vi "Format Data to Save.vi"(5 "Sections":i32=100, 6 "FilePath":path, 7 "LoopBeginWait(ms)":u32=100, 9 "Time":dbl[](array[numeric]), 11 "Data":dbl[][](array[numeric])) -> ()   [LabVIEW 2018]
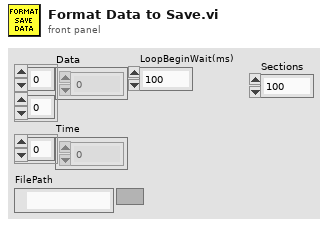
[diagram p1: front panel]
types:
  T1 = enum16{"open", "replace", "create", "open or create", "replace or create", "replace or create with confirmation"}
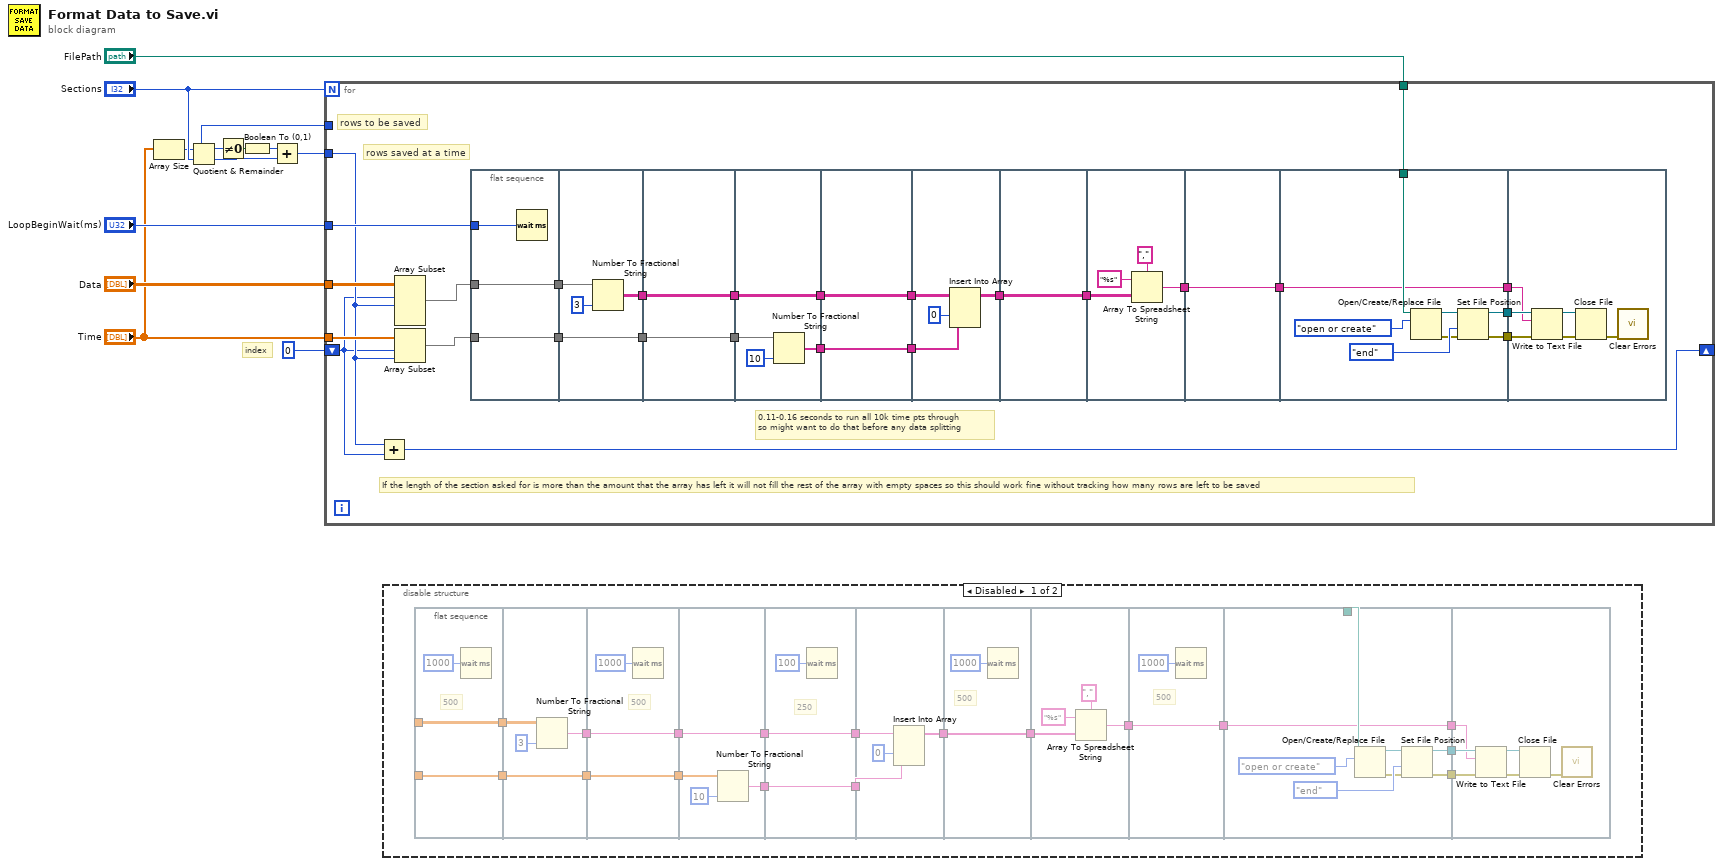
[diagram p0: block diagram]
diagram:
  # "index"
  n1 = Array Size(array="Time") -> (size(s)=w2:i32)
  n2 = Quotient & Remainder(x=w2, y="Sections") -> (x-y*floor(x/y)=w4:i32, floor(x/y)=w5:i32)
  n3 = Not Equal To 0?(x=w4) -> (x != 0?=w7:bool)
  n4 = Boolean To (0,1)(Boolean=w7) -> (0, 1=w6:i16)
  n5 = Add(x=w6, y=w5) -> (x+y=w3:i32)
  n6 = for {
    N: "Sections" -> [_]
    tunnel: "Time" -> [w18]
    tunnel: "Data" -> [w19]
    tunnel: "FilePath" -> [w21]
    tunnel: "LoopBeginWait(ms)" -> [w20]
    tunnel: w3 -> [w14]
    tunnel: w2 -> [_]
    shift-right: [w15] -> _
    shift-left: 0 -> [w13]
    # "rows saved at a time"
    # "rows to be saved"
    # "If the length of the section asked for is more than the amount that the array has left it will not fill the rest of the array with empty spaces so this should work fine without tracking how many rows are left to be saved"
    # "0.11-0.16 seconds to run all 10k time pts through\nso might want to do that before any data splitting"
    n7 = Add(x=w14, y=w13) -> (x+y=w15:i32)
    n8 = Array Subset(array=w19, index (row)=w13, length (row)=w14) -> (w16:dbl[][])  [unwired: 2 in]
    n9 = Array Subset(array=w18, index=w13, length=w14) -> (w17:dbl[])
    n10 = flat-sequence {
      tunnel: w16 -> [w40]
      tunnel: w17 -> [w41]
      tunnel: [w41] -> w38
      tunnel: [w40] -> w37
      tunnel: w20 -> [w39]
      tunnel: w38 -> [w43]
      tunnel: w37 -> [w44]
      tunnel: [w43] -> w36
      tunnel: [w42] -> w35
      tunnel: [w47] -> w34
      tunnel: w36 -> [w47]
      tunnel: w35 -> [w46]
      tunnel: [w46] -> w33
      tunnel: w34 -> [w50]
      tunnel: [w49] -> w32
      tunnel: [w48] -> w31
      tunnel: w33 -> [w48]
      tunnel: w32 -> [w53]
      tunnel: w31 -> [w52]
      tunnel: [w52] -> w30
      tunnel: [w53] -> w29
      tunnel: w30 -> [w56]
      tunnel: w29 -> [w55]
      tunnel: [w54] -> w28
      tunnel: w28 -> [w58]
      tunnel: [w58] -> w27
      tunnel: w27 -> [w60]
      tunnel: [w59] -> w26
      tunnel: w26 -> [w63]
      tunnel: [w63] -> w25
      tunnel: w25 -> [w64]
      tunnel: w21 -> [w67]
      tunnel: [w66] -> w24
      tunnel: [w65] -> w23
      tunnel: [w64] -> w22
      tunnel: w24 -> [w74]
      tunnel: w23 -> [w73]
      tunnel: w22 -> [w72]
      frame #0 {
        n11 = Wait (ms)(milliseconds to wait=w39) -> ()  [unwired: 1 out]
      }
      frame #1 {
        n12 = Number To Fractional String(number=w44, precision (6)=i16 3) -> (F-format string=w42:string[][])  [unwired: 2 in]
      }
      frame #2 {
      }
      frame #3 {
        n13 = Number To Fractional String(number=w50, precision (6)=i16 10) -> (F-format string=w49:string[])  [unwired: 2 in]
      }
      frame #4 {
      }
      frame #5 {
        n14 = Insert Into Array(array=w56, index (col)=0 ("disabled index (col)"), new element=w55) -> (w54:string[][])  [unwired: 1 in]
      }
      frame #6 {
      }
      frame #7 {
        n15 = Array To Spreadsheet String(delimiter (Tab)=",", array=w60, 3:"%s" ("format string")) -> (spreadsheet string=w59:string)
      }
      frame #8 {
      }
      frame #9 {
        n16 = Open/Create/Replace File(file path (use dialog)=w67, operation (0:open)=T1."open or create") -> (refnum out=w69:refnum<file>, error out=w70:errorcluster)  [unwired: 4 in, 1 out]
        n17 = Set File Position(refnum=w69, from (0:start)=enum16{"start", "end", "current"}."end", error in=w70) -> (refnum out=w66:refnum<file>, error out=w65:errorcluster)  [unwired: 1 in]
      }
      frame #10 {
        n18 = Write to Text File(file (use dialog)=w74, text=w72, error in=w73) -> (refnum out=w76:refnum<file>, error out=w75:errorcluster)  [unwired: 1 in, 1 out]
        n19 = Close File(refnum=w76, error in=w75) -> (error out=w77:errorcluster)  [unwired: 1 out]
        n20 = call <vilib>:"Clear Errors.vi"("error in (no error)"=w77) -> ()  [unwired: 5 in, 2 out]
      }
    }
  }
  n21 = disable-structure shown="Disabled" {
    frame Disabled {
      n22 = flat-sequence {
        tunnel: _ -> [w96]
        tunnel: _ -> [w97]
        tunnel: [w97] -> w94
        tunnel: [w96] -> w93
        tunnel: w94 -> [w99]
        tunnel: w93 -> [w100]
        tunnel: [w99] -> w92
        tunnel: [w98] -> w91
        tunnel: [w104] -> w90
        tunnel: w92 -> [w104]
        tunnel: w91 -> [w102]
        tunnel: [w102] -> w89
        tunnel: w90 -> [w107]
        tunnel: [w106] -> w88
        tunnel: [w105] -> w87
        tunnel: w89 -> [w105]
        tunnel: w88 -> [w111]
        tunnel: w87 -> [w110]
        tunnel: [w110] -> w86
        tunnel: [w111] -> w85
        tunnel: w86 -> [w114]
        tunnel: w85 -> [w113]
        tunnel: [w112] -> w84
        tunnel: w84 -> [w117]
        tunnel: [w117] -> w83
        tunnel: w83 -> [w119]
        tunnel: [w118] -> w82
        tunnel: w82 -> [w123]
        tunnel: [w123] -> w81
        tunnel: w81 -> [w124]
        tunnel: _ -> [w127]
        tunnel: [w126] -> w80
        tunnel: [w125] -> w79
        tunnel: [w124] -> w78
        tunnel: w80 -> [w134]
        tunnel: w79 -> [w133]
        tunnel: w78 -> [w132]
        frame #0 {
          # "500"
          n23 = Wait (ms)(milliseconds to wait=u32 1000) -> ()  [unwired: 1 out]
        }
        frame #1 {
          n24 = Number To Fractional String(number=w100, precision (6)=i16 3) -> (F-format string=w98:string)  [unwired: 2 in]
        }
        frame #2 {
          # "500"
          n25 = Wait (ms)(milliseconds to wait=u32 1000) -> ()  [unwired: 1 out]
        }
        frame #3 {
          n26 = Number To Fractional String(number=w107, precision (6)=i16 10) -> (F-format string=w106:string)  [unwired: 2 in]
        }
        frame #4 {
          # "250"
          n27 = Wait (ms)(milliseconds to wait=u32 100) -> ()  [unwired: 1 out]
        }
        frame #5 {
          n28 = Insert Into Array(array=w114, index (col)=0 ("disabled index (col)"), new element=w113) -> (w112:string[])  [unwired: 1 in]
        }
        frame #6 {
          # "500"
          n29 = Wait (ms)(milliseconds to wait=u32 1000) -> ()  [unwired: 1 out]
        }
        frame #7 {
          n30 = Array To Spreadsheet String(delimiter (Tab)=",", array=w119, 3:"%s" ("format string")) -> (spreadsheet string=w118:string)
        }
        frame #8 {
          # "500"
          n31 = Wait (ms)(milliseconds to wait=u32 1000) -> ()  [unwired: 1 out]
        }
        frame #9 {
          n32 = Open/Create/Replace File(file path (use dialog)=w127, operation (0:open)=T1."open or create") -> (refnum out=w129:refnum<file>, error out=w130:errorcluster)  [unwired: 4 in, 1 out]
          n33 = Set File Position(refnum=w129, from (0:start)=enum16{"start", "end", "current"}."end", error in=w130) -> (refnum out=w126:refnum<file>, error out=w125:errorcluster)  [unwired: 1 in]
        }
        frame #10 {
          n34 = Write to Text File(file (use dialog)=w134, text=w132, error in=w133) -> (refnum out=w136:refnum<file>, error out=w135:errorcluster)  [unwired: 1 in, 1 out]
          n35 = Close File(refnum=w136, error in=w135) -> (error out=w137:errorcluster)  [unwired: 1 out]
          n36 = call <vilib>:"Clear Errors.vi"("error in (no error)"=w137) -> ()  [unwired: 5 in, 2 out]
        }
      }
    }
    frame Enabled {
    }
  }
